vi "Execute Process Step.vi"(8 "error in (no error)":errorcluster, 11 "Process Model in":refnum<class "Process Model.lvclass">) -> (0 "error out":errorcluster, 3 "Process Model out":refnum<class "Process Model.lvclass">)   [LabVIEW 2019, in "Process Model.lvclass"]
uses:
  <vilib>/gpm_packages/@cs/Car-wash/Source/Process Model/Process Model.lvclass
  C:/Program Files/National Instruments/LabVIEW 2019/vi.lib/ActorFramework/Actor/Actor.lvclass
  <vilib>/gpm_packages/@cs/Car-wash/Source/Process Model/Process Model.lvclass/Process Model.ctl
  <vilib>/gpm_packages/@cs/Car-wash/Source/iProcess Step Model/iProcess Step Model/iProcess Step Model.lvclass
  C:/Program Files/National Instruments/LabVIEW 2019/vi.lib/gpm_packages/@cs/mva-core/Source/IModel/IModel/IModel.lvclass
  <vilib>/ActorFramework/Message Enqueuer/Message Enqueuer.lvclass/Message Enqueuer.ctl
  <vilib>/ActorFramework/Actor/Actor.lvclass/Actor.ctl
  <vilib>/ActorFramework/Message Enqueuer/Enqueue.vi
  <vilib>/ActorFramework/Message Enqueuer/Init from Existing Queue.vi
  <vilib>/gpm_packages/@cs/Car-wash/Source/iProcess Step Model/iProcess Step Model Messages/Execute Msg/Execute Msg.lvclass
  C:/Program Files/National Instruments/LabVIEW 2019/vi.lib/ActorFramework/Message/Message.lvclass
  <vilib>/gpm_packages/@cs/Car-wash/Source/iProcess Model/iProcess Model Messages/Stop Process Msg/Stop Process Msg.lvclass
  <vilib>/ActorFramework/Message Priority Queue/Priority Enqueue.vi
  <vilib>/ActorFramework/Message Enqueuer/Message Enqueuer.lvclass
  <vilib>/gpm_packages/@cs/test-executive/Source/Test Executive/TestExecutive Ref/TestExecutive Ref.lvclass
  <vilib>/ActorFramework/Actor/Actor.lvclass
  <vilib>/gpm_packages/@cs/test-executive/Source/Test Executive/Executioner/Executioner.lvclass
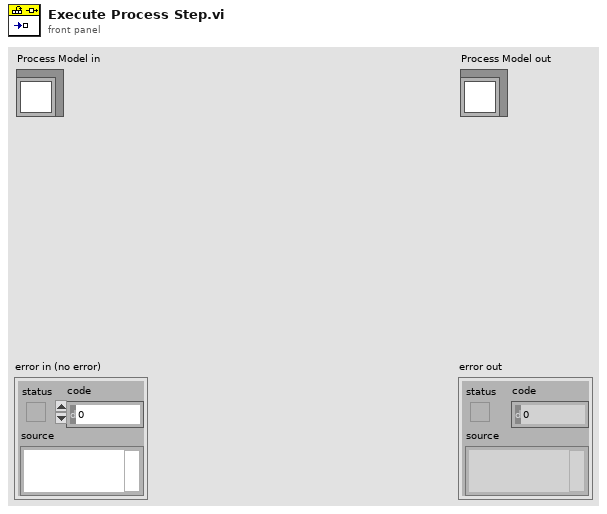
[diagram p1: front panel]
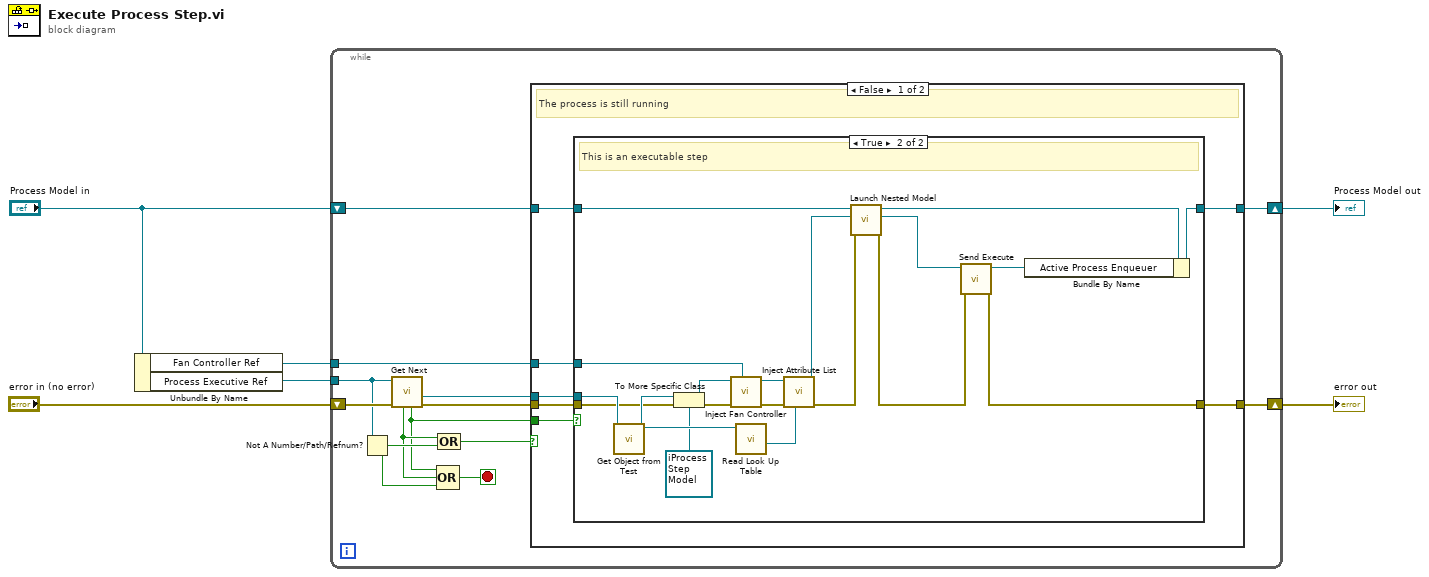
[diagram p0: block diagram]
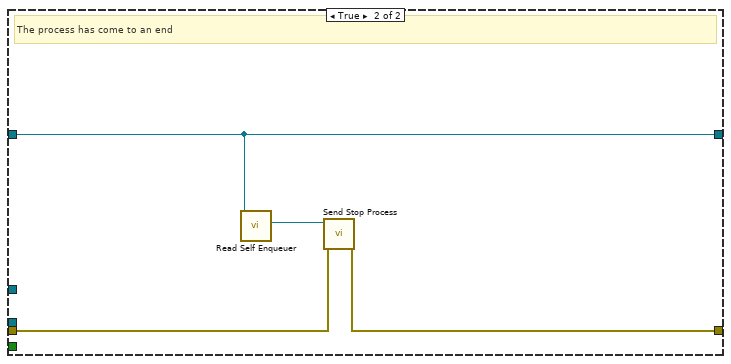
[diagram p3: hidden frame]
diagram:
  n1 = Unbundle By Name("Process Model in") -> ("Fan Controller Ref"=w1:refnum<data-value>, "Process Executive Ref"=w2:refnum<data-value>)
  n2 = while {
    shift-right: [w15] -> w6
    shift-left: "Process Model in" -> [w16]
    shift-right: [w13] -> w4
    shift-left: "error in (no error)" -> [w19]
    tunnel: w2 -> [w18]
    tunnel: w1 -> [w7]
    stop <- w17 stop-if-true
    n3 = Not A Number/Path/Refnum?(number/path/refnum=w18) -> (NaN/Path/Refnum?=w12:bool)
    n4 = call <vilib>:"Get Next.vi"("error in (no error)"=w19, "Test Executive Ref"=w18) -> ("error out"=w14:errorcluster, "Test"=w9:refnum<class "Executioner.lvclass">, "Found"=w8:bool, "Complete"=w11:bool)  [unwired: 3 in, 3 out]
    n5 = Compound Arithmetic op=OR(w8, w11, w12) -> (w17:bool)
    n6 = Compound Arithmetic op=OR(w11, w12) -> (w10:bool)
    n7 = case shown="False" w10 {
      tunnel: [w24 w52] -> w15
      tunnel: w16 -> [w25 w52]
      tunnel: [w22 w49] -> w13
      tunnel: w14 -> [w23 w50]
      tunnel: w9 -> [w21 _]
      tunnel: w8 -> [w26 _]
      tunnel: w7 -> [w20 _]
      frame False {
        # "The process is still running"
        n8 = case shown="True" w26 {
          tunnel: [w28 w38] -> w24
          tunnel: w25 -> [w28 w42]
          tunnel: [w27 w34] -> w22
          tunnel: w23 -> [w27 w45]
          tunnel: w21 -> [_ w48]
          tunnel: w20 -> [_ w29]
          frame False {
            # "This is a flow control process"
          }
          frame True {
            # "This is an executable step"
            n9 = call <vilib>:"Get Object from Test.vi"("Executioner in"=w48) -> ("Test"=w46:refnum<class>, "Executioner out"=w47:refnum<class "Executioner.lvclass">)  [unwired: 9 in]
            n10 = To More Specific Class(target class=refnum<class "iProcess Step Model.lvclass"> refnum ("iProcess Step Model.lvclass"), reference=w46, error in=w45) -> (specific class reference=w31:refnum<class "iProcess Step Model.lvclass">, error out=w33:errorcluster)
            n11 = call-dynamic "Inject Fan Controller.vi"("Fan Controller Ref"=w29, "error in (no error)"=w33, "iProcess Step Model in"=w31) -> ("error out"=w32:errorcluster, "iProcess Step Model out"=w30:refnum<class "iProcess Step Model.lvclass">)  [unwired: 7 in]
            n12 = call <vilib>:"Read Look Up Table.vi"("Executioner in"=w47) -> ("Attributes Ref"=w43:refnum<data-value>)  [unwired: 9 in, 1 out]
            n13 = call-dynamic "Inject Attribute List.vi"("Attributes Ref"=w43, "error in (no error)"=w32, "iProcess Step Model in"=w30) -> ("error out"=w41:errorcluster, "iProcess Step Model out"=w40:refnum<class "iProcess Step Model.lvclass">)  [unwired: 7 in]
            n14 = call-dynamic "Launch Nested Model.vi"("error in (no error)"=w41, "Model to Launch"=w40, "IModel in"=w42) -> ("error out"=w35:errorcluster, "Nested Model Enqueuer"=w37:refnum<class "Message Enqueuer.lvclass">, "IModel out"=w39:refnum<class "Process Model.lvclass">)  [unwired: 6 in]
            n15 = call <vilib>:"Send Execute.vi"("error in (no error)"=w35, "Message Enqueuer"=w37) -> ("error out"=w34:errorcluster, "Message Enqueuer out"=w36:refnum<class "Message Enqueuer.lvclass">)  [unwired: 8 in]
            n16 = Bundle By Name(cluster=w39, "Active Process Enqueuer"=w36) -> (w38:refnum<class "Process Model.lvclass">)
          }
        }
      }
      frame True {
        # "The process has come to an end"
        n17 = call <vilib>:"Read Self Enqueuer.vi"("Actor"=w52) -> ("Self Enqueuer"=w51:refnum<class "Message Enqueuer.lvclass">)  [unwired: 10 in]
        n18 = call <vilib>:"Send Stop Process.vi"("error in (no error)"=w50, "Message Enqueuer"=w51) -> ("error out"=w49:errorcluster)  [unwired: 8 in, 1 out]
      }
    }
  }
  "error out" <- w4
  "Process Model out" <- w6
